vi "FM Receiver.vi"() -> ()   [LabVIEW 2013]
doc: "Use this template to build a producer/consumer design pattern. Use this template when you need to execute a process, such as data analysis, when a data source, such as a triggered acquisition, produces data at an uneven rate and you need to execute the process when the data becomes available."
uses:
  <vilib>/sound2/lvsound2.llb/Sound Output Write (DBL Single).vi
  <vilib>/Analysis/2dsp.llb/Rational Resample (single channel, DBL).vi
  <vilib>/Waveform/WDTFileIO.llb/Read Waveform from File.vi
  <vilib>/Analysis/NI_AALPro.lvlib
panel:
  out "time":string
  out "date":string
  out "XY Graph":cdb[](graph)
  in  "Name":cluster{"Decimation":u32, "Interpolation":u32}
  out "error out":errorcluster
  in  "Sound format":T1
  in  "IQ Rate":u32
  out "Waveform":waveform(dbl)(graph)
  out "error out":errorcluster
  in  "file path (dialog if empty)":path
  in  "stop":bool
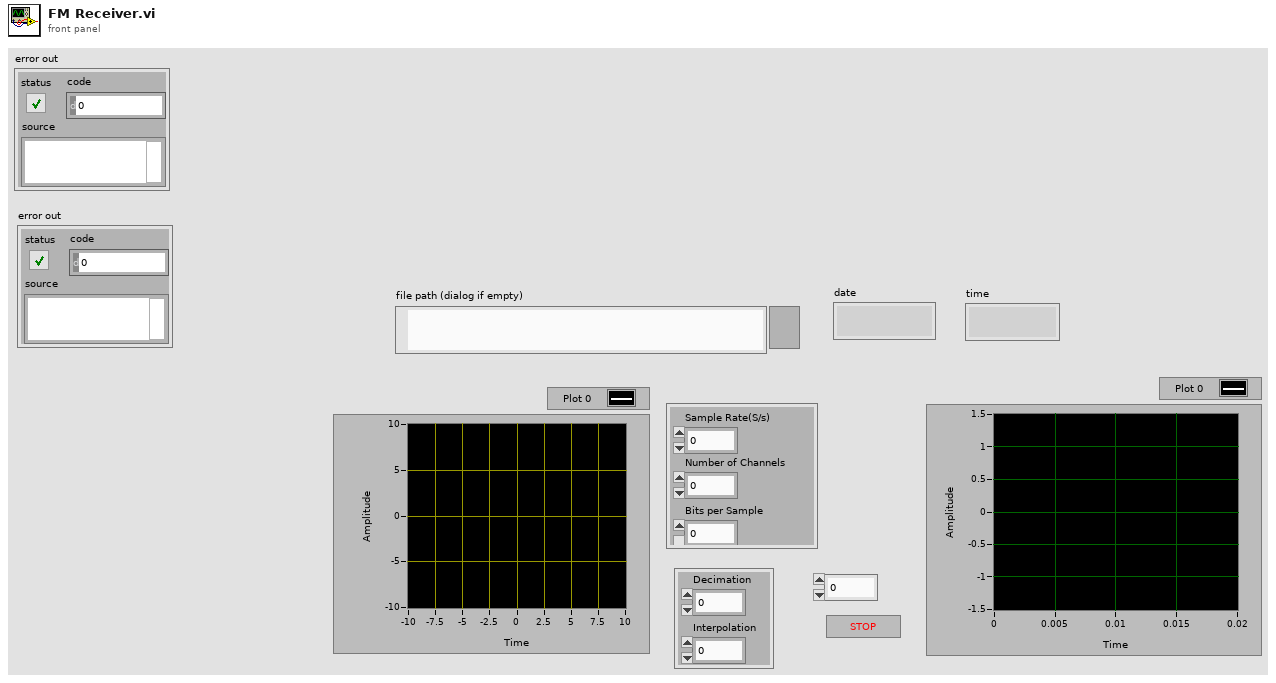
[diagram p1: front panel]
types:
  T1 = cluster{"Sample Rate(S/s)":dbl, "Number of Channels":dbl, "Bits per Sample":dbl}
  T2 = typedef "Sound Output Task ID.ctl" = u32
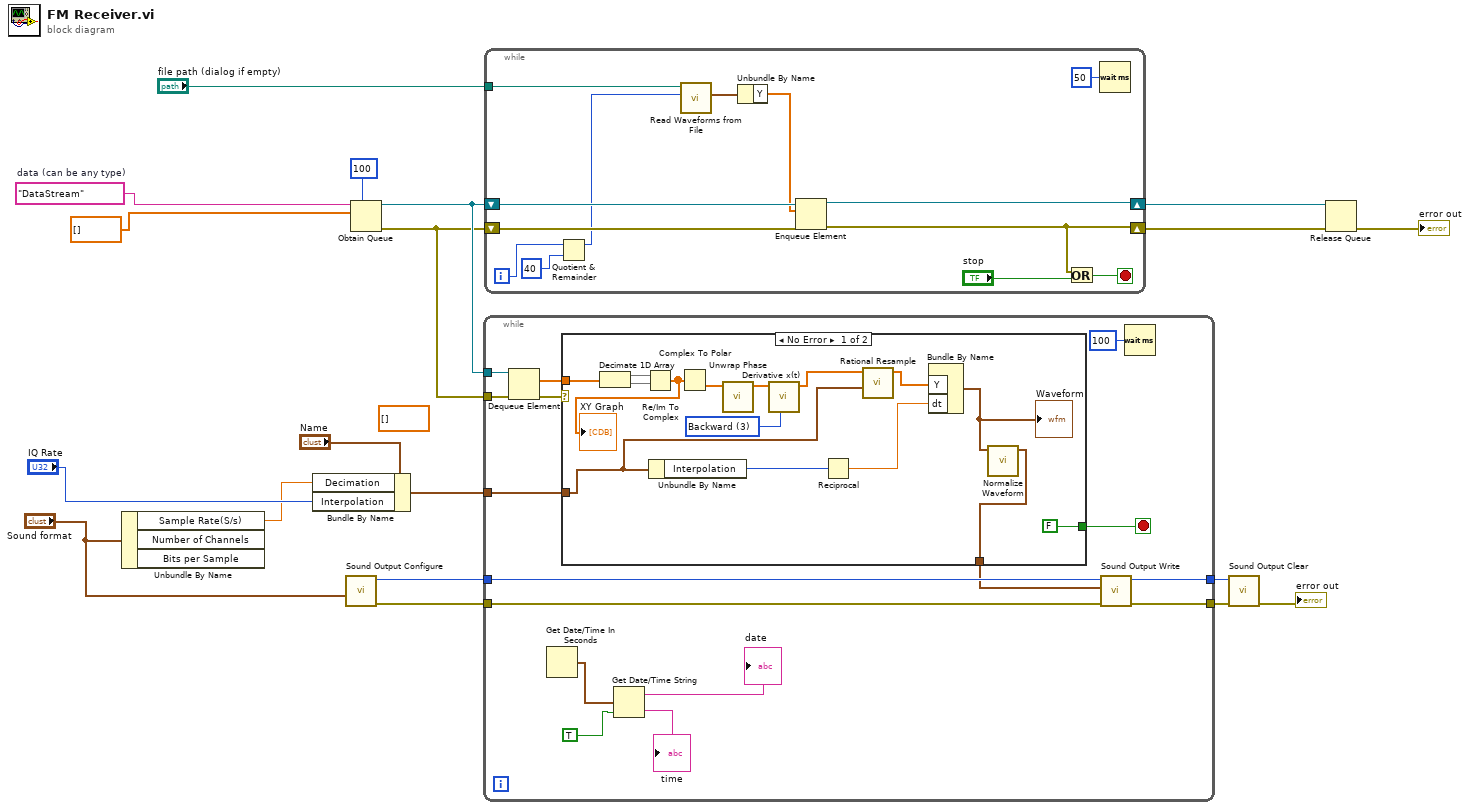
[diagram p0: block diagram]
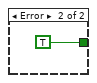
[diagram p2: hidden frame]
diagram:
  (unwired) dbl[] []
  w12 = "DataStream"  # data (can be any type)
  n1 = Unbundle By Name("Sound format") -> ("Sample Rate(S/s)"=w2:dbl)  [unwired: 2 out]
  n2 = Bundle By Name(cluster="Name", "Decimation"=w2, "Interpolation"="IQ Rate") -> (w4:cluster{"Decimation":u32, "Interpolation":u32})
  n3 = call <vilib>:"Sound Output Configure.vi"("sound format"="Sound format") -> ("error out"=w8:errorcluster, "task ID"=w6:T2)  [unwired: 9 in]
  n4 = Obtain Queue(max queue size (-1, unlimited)=100, name (unnamed)=w12, element data type=dbl[] []) -> (queue out=w19:refnum<queue>, error out=w13:errorcluster)  [unwired: 2 in, 1 out]
  n5 = while {
    tunnel: w19 -> [w35]
    tunnel: w13 -> [w31]
    tunnel: [w29] -> w10
    tunnel: [w28] -> w9
    tunnel: w8 -> [w27]
    tunnel: w6 -> [w26]
    tunnel: w4 -> [w24]
    stop <- w32 stop-if-true
    n6 = Dequeue Element(queue=w35, error in (no error)=w31) -> (element=w33:dbl[], error out=w34:errorcluster)  [unwired: 1 in, 2 out]
    n7 = Get Date/Time In Seconds() -> (seconds since 1Jan1904=w23:timestamp)
    n8 = case shown="No Error" w34 {
      tunnel: w33 -> [w49 _]
      tunnel: [FALSE TRUE] -> w32
      tunnel: [w38 _] -> w25
      tunnel: w24 -> [w47 _]
      frame No Error {
        w37 = u16 3 items=["2nd Order Central", "4th Order Central", "Forward", "Backward"] ("method")
        n9 = Decimate 1D Array(w49) -> (w45:dbl[], w44:dbl[])
        n10 = Re/Im To Complex(1:w44, 2:w45) -> (0:w36:cdb[])
        "XY Graph" <- w36
        n11 = Unbundle By Name(w47) -> ("Interpolation"=w46:u32)
        n12 = Complex To Polar(r * e^(i*theta)=w36) -> (theta=w43:dbl[])  [unwired: 1 out]
        n13 = call <vilib>:"Unwrap Phase.vi"("Phase"=w43) -> ("Unwrapped Phase"=w41:dbl[])  [unwired: 9 in, 1 out]
        n14 = call <vilib>:"Derivative x(t).vi"("method"=w37, "X"=w41) -> ("dX/dt"=w40:dbl[])  [unwired: 8 in, 1 out]
        n15 = Reciprocal(x=w46) -> (1/x=w48:dbl)
        n16 = call-poly <vilib>:"Rational Resample.vi"("resample factor"=w47, "X"=w40) -> ("Y"=w42:dbl[])  [unwired: 7 in, 2 out]
        n17 = Bundle By Name("Y"=w42, "dt"=w48) -> (w39:waveform(dbl))  [unwired: 1 in]
        "Waveform" <- w39
        n18 = call <vilib>:"Normalize Waveform.vi"("waveform in"=w39) -> ("normalized waveform"=w38:waveform(dbl))  [unwired: 7 in, 3 out]
      }
      frame Error {
      }
    }
    n19 = Get Date/Time String(seconds (now)=w23, want seconds? (F)=TRUE) -> (date string=→"date":string, time string=→"time":string)  [unwired: 1 in]
    n20 = call-poly <vilib>:"Sound Output Write.vi"("error in (no error)"=w27, "data"=w25, "task ID"=w26) -> ("error out"=w28:errorcluster, "task ID out"=w29:T2)  [unwired: 7 in]
    n21 = Wait (ms)(milliseconds to wait=u32 100) -> ()  [unwired: 1 out]
  }
  n22 = while {
    shift-right: [w53] -> w17
    shift-left: w13 -> [w60]
    shift-right: [w61] -> w18
    shift-left: w19 -> [w59]
    tunnel: "file path (dialog if empty)" -> [w63]
    i -> [w58]
    stop <- w54 stop-if-true
    n23 = Quotient & Remainder(x=w58, y=40) -> (x-y*floor(x/y)=w56:i32)  [unwired: 1 out]
    n24 = call-poly <vilib>:"Read Waveforms from File.vi"("offset (records:0)"=w56, "file path (dialog if empty)"=w63) -> ("first waveform in record"=w62:waveform(dbl))  [unwired: 4 in, 3 out]
    n25 = Unbundle By Name(w62) -> ("Y"=w55:dbl[])
    n26 = Enqueue Element(queue=w59, element=w55, error in (no error)=w60) -> (queue out=w61:refnum<queue>, error out=w53:errorcluster)  [unwired: 1 in, 1 out]
    n27 = Or(x=w53, y="stop") -> (x .or. y?=w54:bool)
    n28 = Wait (ms)(milliseconds to wait=u32 50) -> ()  [unwired: 1 out]
  }
  n29 = call <vilib>:"Sound Output Clear.vi"("error in (no error)"=w9, "task ID"=w10) -> ("error out"=→"error out":errorcluster)  [unwired: 9 in]
  n30 = Release Queue(queue=w18, error in (no error)=w17) -> (error out=→"error out":errorcluster)  [unwired: 1 in, 2 out]
